vi "Build Driver Settings Mappings.vi"(8 "error in (no error)":errorcluster, 11 "Pico in":refnum<class "Pico.lvclass">) -> (0 "error out":errorcluster, 3 "Pico out":refnum<class "Pico.lvclass">)   [LabVIEW 2023, in "HAF.lvlib" / "Pico.lvclass"]
uses:
  Pico.lvclass
  Pico.lvclass/Pico.ctl
  Driver/Driver.lvclass
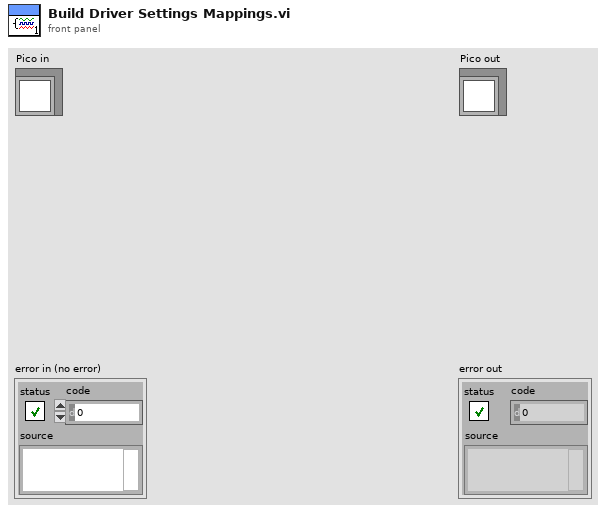
[diagram p1: front panel]
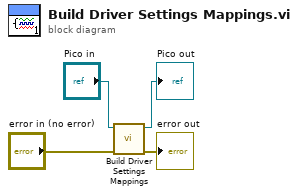
[diagram p0: block diagram]
diagram:
  n1 = call-parent "Build Driver Settings Mappings.vi"("error in (no error)"="error in (no error)", "Driver in"="Pico in") -> ("error out"=→"error out":errorcluster, "Driver out"=→"Pico out":refnum<class "Pico.lvclass">)  [unwired: 8 in]
